vi "Convert to Kabab Case.vi"(8 "error in (no error)":errorcluster, 11 "Input String":string) -> (0 "error out":errorcluster, 3 "Output String":string)   [LabVIEW 2015, in "Case Manipulation.lvlib"]
doc: "Introduction:\nWe often remove the spaces between words because programs of different sorts reserve the space (‘ ’) character for special purposes. Because the space character is reserved, we cannot use it to represent a concept that we express in our human language with multiple words.\nKabab Case:\nThis style is often used in URLs. For example, www.blog.com/cool-article-1. It is a nice, clean, human-readable way to combine the words."
uses:
  Case Manipulation.lvlib
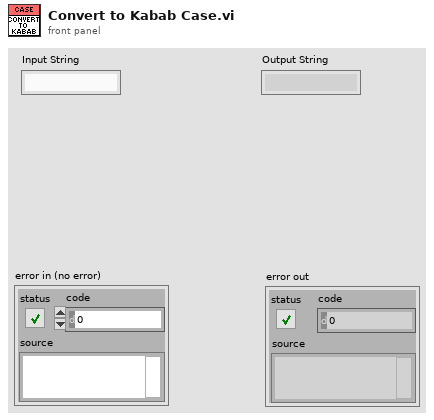
[diagram p1: front panel]
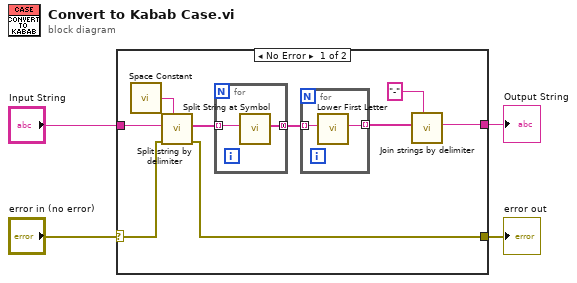
[diagram p0: block diagram]
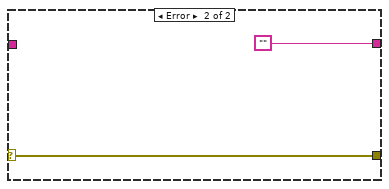
[diagram p2: hidden frame]
diagram:
  n1 = case shown="No Error" "error in (no error)" {
    selector: "error in (no error)" -> [w11 w19]
    tunnel: "Input String" -> [w13 _]
    tunnel: [w10 w19] -> w2
    tunnel: [w7 ""] -> w1
    frame No Error {
      n2 = call <vilib>:"Space Constant.vi"() -> ("String"=w12:string)
      n3 = call "Split string by delimiter.vi"("Delimiter"=w12, "error in (no error)"=w11, "String In"=w13) -> ("error out"=w10:errorcluster, "String Array Out"=w6:string[])  [unwired: 7 in]
      n4 = for {
        tunnel: w6 -> [w15] mode=indexing
        tunnel: [w14] -> w5 mode=concatenating
        n5 = call "Split String at Symbol.vi"("String In"=w15) -> ("String Array Out"=w14:string[])  [unwired: 9 in, 1 out]
      }
      n6 = for {
        tunnel: w5 -> [w17] mode=indexing
        tunnel: [w16] -> w9 mode=indexing
        n7 = call "Lower First Letter.vi"("String In"=w17) -> ("String Out"=w16:string)  [unwired: 10 in]
      }
      n8 = call "Join strings by delimiter.vi"("Delimiter"="-", "Strings []"=w9) -> ("String Out"=w7:string)  [unwired: 9 in]
    }
    frame Error {
    }
  }
  "error out" <- w2
  "Output String" <- w1
